vi "Dequeue.vi"(8 "Error In":errorcluster, 9 "timeout in ms (-1)":i32=-1, 11 "queue in":refnum<queue>) -> (0 "Error Out":errorcluster, 1 "Data":variant, 2 "Message":string, 3 "queue out":refnum<queue>)   [LabVIEW 2019, in "Queue.lvlib"]
uses:
  Queue.lvlib
  Message Cluster.ctl
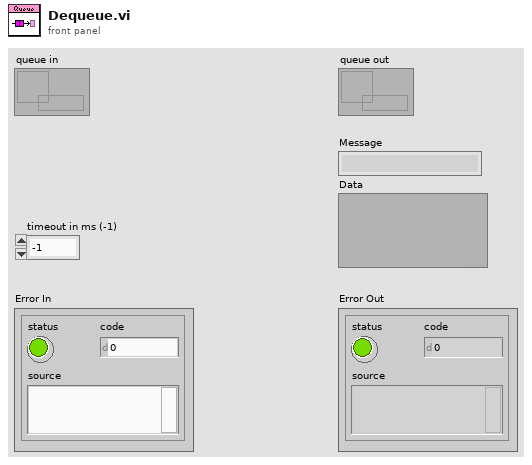
[diagram p1: front panel]
types:
  T1 = typedef "Queue.lvlib/Message Cluster.ctl" = cluster{"Message":string, "Data":variant}
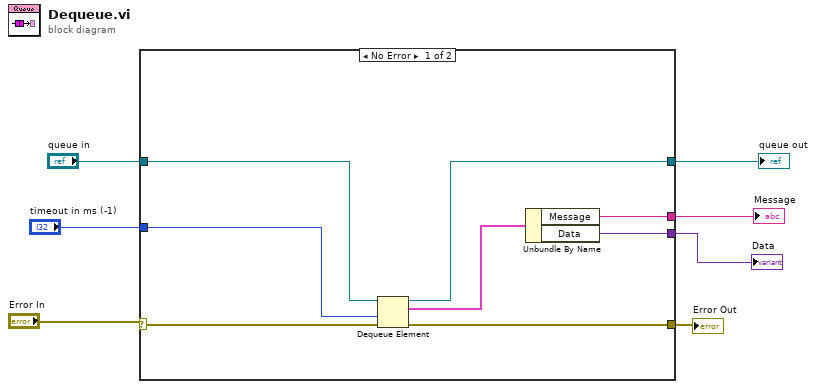
[diagram p0: block diagram]
diagram:
  n1 = case shown="No Error" "Error In" {
    selector: "Error In" -> [w15 w17]
    tunnel: [w14 w17] -> w6
    tunnel: [w13 w16] -> w5
    tunnel: "queue in" -> [w12 w16]
    tunnel: [w10 _] -> w3
    tunnel: [w9 _] -> w2
    tunnel: "timeout in ms (-1)" -> [w8 _]
    frame No Error {
      n2 = Dequeue Element(queue=w12, timeout in ms (-1)=w8, error in (no error)=w15) -> (queue out=w13:refnum<queue>, element=w11:T1, error out=w14:errorcluster)  [unwired: 1 out]
      n3 = Unbundle By Name(w11) -> ("Message"=w10:string, "Data"=w9:variant)
    }
    frame Error {
    }
  }
  "Error Out" <- w6
  "queue out" <- w5
  "Message" <- w3
  "Data" <- w2
